vi "LV to DAT.vi"   [LabVIEW 2016, in "LV to ITX.lvclass"]
uses:
  LV to ITX.lvclass
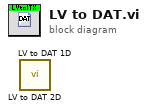
[diagram p0: block diagram]
diagram:
  n1 = call "LV to DAT 2D.vi"() -> ()  [unwired: 10 in, 2 out]
  n2 = call "LV to DAT 1D.vi"() -> ()  [unwired: 10 in, 2 out]
